vi "DBL Array to Result.vi"(7 "Result name":string, 8 "Error In":errorcluster, 10 "Data":dbl[](array[numeric]), 11 "Channel Names":string[](array[string])) -> (0 "Error Out":errorcluster, 3 "Mag Lab Result out":refnum<class "Mag Lab Result.lvclass">)   [LabVIEW 2015]
uses:
  Mag Lab Result.lvclass
  Waveform Array Result/Waveform Array Result.lvclass
  Mag Lab Result.lvclass/Mag Lab Result.ctl
  Waveform Array Result/Waveform Array Result.lvclass/Waveform Array Result.ctl
  Write Group Name.vi
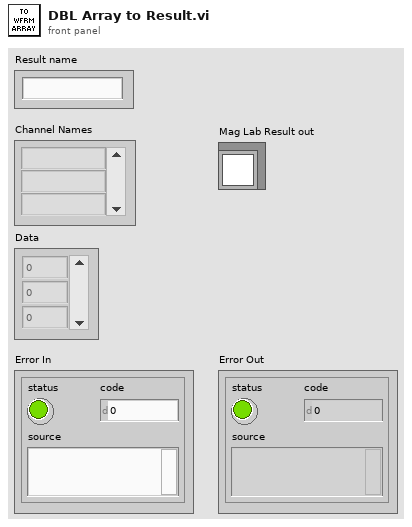
[diagram p1: front panel]
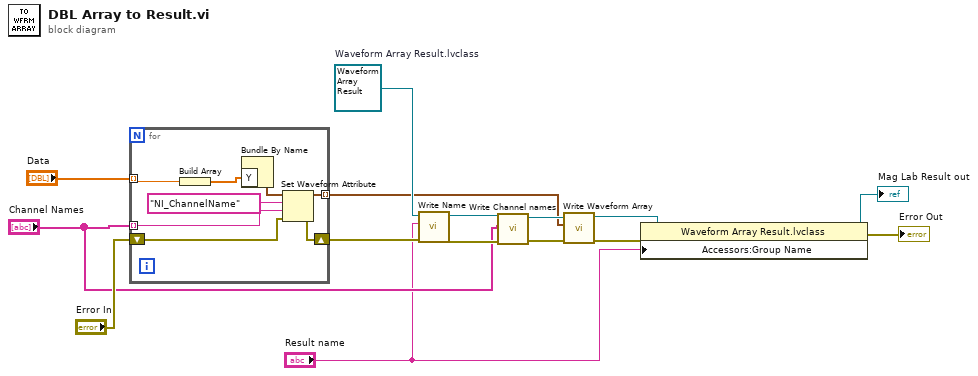
[diagram p0: block diagram]
diagram:
  w13 = refnum<class "Waveform Array Result.lvclass"> refnum  # Waveform Array Result.lvclass
  n1 = for {
    tunnel: "Data" -> [w23] mode=indexing
    tunnel: "Channel Names" -> [w19] mode=indexing
    shift-right: [w17] -> w12
    shift-left: "Error In" -> [w18]
    tunnel: [w16] -> w6 mode=indexing
    n2 = Build Array(w23) -> (w22:dbl[])
    n3 = Bundle By Name("Y"=w22) -> (w21:waveform(dbl))  [unwired: 1 in]
    n4 = Set Waveform Attribute(4:w18, 5:w19, 6:"NI_ChannelName", 7:w21) -> (0:w17:errorcluster, 3:w16:waveform(dbl))  [unwired: 1 out]
  }
  n5 = call "Write Name.vi"("error in (no error)"=w12, "Name"="Result name", "Mag Lab Result in"=w13) -> ("error out"=w11:errorcluster, "Mag Lab Result out"=w10:refnum<class "Waveform Array Result.lvclass">)  [unwired: 7 in]
  n6 = call "Write Channel names.vi"("error in (no error)"=w11, "Channel names"="Channel Names", "Waveform Array Result in"=w10) -> ("error out"=w8:errorcluster, "Waveform Array Result out"=w7:refnum<class "Waveform Array Result.lvclass">)  [unwired: 7 in]
  n7 = call "Write Waveform Array.vi"("error in (no error)"=w8, "Waveform Array"=w6, "Waveform Array Result in"=w7) -> ("error out"=w3:errorcluster, "Waveform Array Result out"=w5:refnum<class "Waveform Array Result.lvclass">)  [unwired: 7 in]
  n8 = property class="Waveform Array Result.lvclass"(reference=w5, error in=w3, "Accessors:Group Name"="Result name") -> (reference out=→"Mag Lab Result out":refnum<class "Waveform Array Result.lvclass">, error out=→"Error Out":errorcluster)
